vi "BuildDestinationExists.vi"(8 "error in (no error)":errorcluster, 11 "ProjectItem in":refnum<class "ProjectItem.lvclass">) -> (0 "error out":errorcluster, 1 "Exists":bool, 2 "path out":path, 3 "ProjectItem out":refnum<class "ProjectItem.lvclass">)   [LabVIEW 2019, in "SolutionBuilder.lvlib" / "ProjectItem.lvclass"]
uses:
  ProjectItem.lvclass
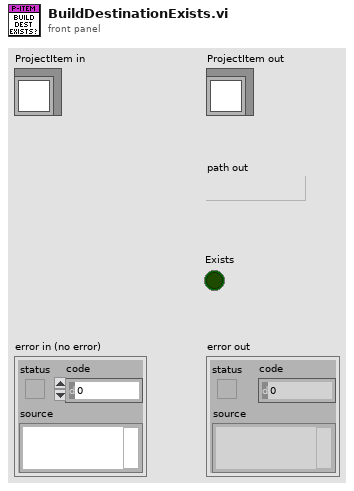
[diagram p1: front panel]
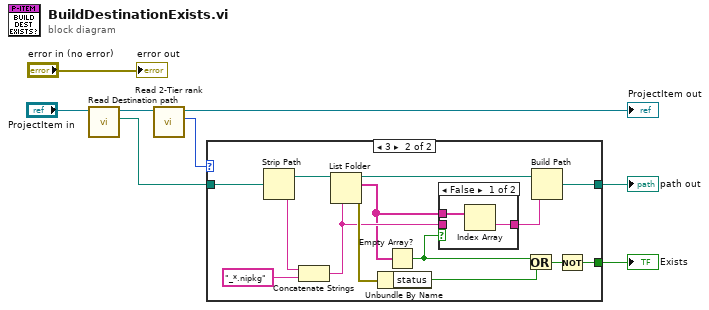
[diagram p0: block diagram]
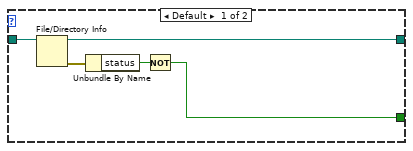
[diagram p2: hidden frame]
diagram:
  n1 = call "Read Destination path.vi"("ProjectItem in"="ProjectItem in") -> ("Destination path"=w5:path, "ProjectItem out"=w6:refnum<class "ProjectItem.lvclass">)  [unwired: 9 in]
  n2 = call "Read 2-Tier rank.vi"("ProjectItem in"=w6) -> ("2-Tier rank"=w7:u8, "ProjectItem out"=→"ProjectItem out":refnum<class "ProjectItem.lvclass">)  [unwired: 9 in]
  n3 = case shown="3" w7 {
    tunnel: w5 -> [w13 w22]
    tunnel: [w10 w20] -> w2
    tunnel: [w9 w16] -> w1
    frame Default {
      n4 = File/Directory Info(path=w13) -> (path out=w9:path, error out=w12:errorcluster)  [unwired: 1 in, 5 out]
      n5 = Unbundle By Name(w12) -> ("status"=w11:bool)
      n6 = Not(x=w11) -> (.not. x?=w10:bool)
    }
    frame 3 {
      n7 = Strip Path(path=w22) -> (stripped path=w27:path, name=w26:string)
      n8 = Concatenate Strings(w26, "_*.nipkg" ("string")) -> (w18:string)
      n9 = List Folder(path=w27, pattern=w18) -> (path out=w17:path, filenames=w14:string[], error out=w24:errorcluster)  [unwired: 2 in, 1 out]
      n10 = Unbundle By Name(w24) -> ("status"=w23:bool)
      n11 = Empty Array?(array=w14) -> (empty?=w19:bool)
      n12 = case shown="False" w19 {
        tunnel: w18 -> [_ w30]
        tunnel: [w28 w30] -> w15
        tunnel: w14 -> [w29 _]
        frame False {
          n13 = Index Array(array=w29) -> (element=w28:string)  [unwired: 1 in]
        }
        frame True {
        }
      }
      n14 = Or(x=w19, y=w23) -> (x .or. y?=w21:bool)
      n15 = Build Path(base path=w17, name or relative path=w15) -> (appended path=w16:path)
      n16 = Not(x=w21) -> (.not. x?=w20:bool)
    }
  }
  "Exists" <- w2
  "path out" <- w1
  "error out" <- "error in (no error)"
